vi "Stop Core Kill Queues.vi"(8 "error in (no error)":errorcluster, 11 "AMS Gas in":refnum<class "AMS Gas.lvclass">) -> (0 "error out":errorcluster, 3 "AMS Gas out":refnum<class "AMS Gas.lvclass">)   [LabVIEW 2015, in "AMS UI.lvlib" / "AMS Gas.lvclass"]
uses:
  AMS Gas.lvclass
  AMS Gas.lvclass/AMS Gas.ctl
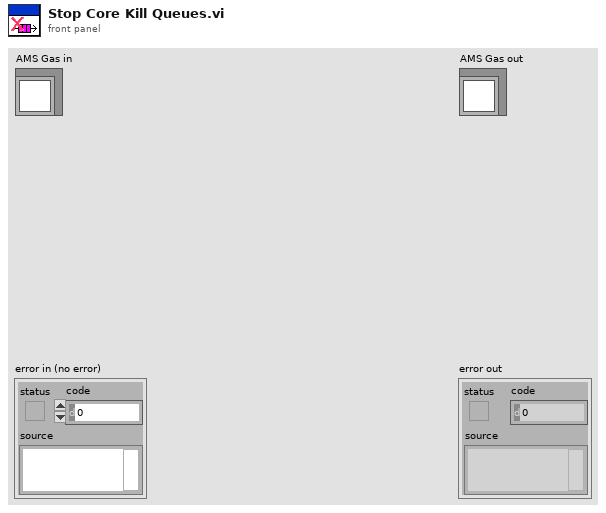
[diagram p1: front panel]
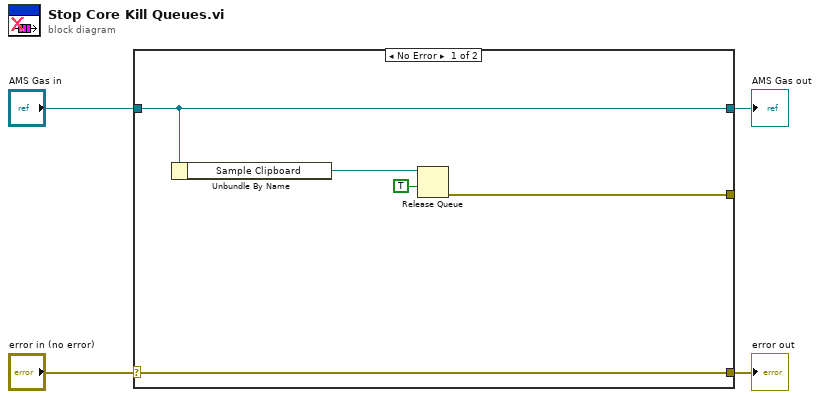
[diagram p0: block diagram]
diagram:
  n1 = case shown="No Error" "error in (no error)" {
    selector: "error in (no error)" -> [w9 w11]
    tunnel: [w9 w11] -> w3
    tunnel: [w8 w10] -> w1
    tunnel: "AMS Gas in" -> [w8 w10]
    tunnel: [w6 _] -> _
    frame No Error {
      n2 = Unbundle By Name(w8) -> ("Sample Clipboard"=w7:refnum<queue>)
      n3 = Release Queue(queue=w7, force destroy? (F)=TRUE) -> (error out=w6:errorcluster)  [unwired: 1 in, 2 out]
    }
    frame Error {
    }
  }
  "error out" <- w3
  "AMS Gas out" <- w1
